vi "setStringValue.vi"(8 "error in (no error)":errorcluster, 10 "stringValue":string, 11 "xmlNode.lvclass in":refnum<class "xmlNode.lvclass">) -> (0 "error out":errorcluster, 3 "xmlNode.lvclass out":refnum<class "xmlNode.lvclass">)   [LabVIEW 2009, in "Tools.lvlib" / "xml.lvlib" / "xmlNode.lvclass"]
doc: "Sets the String value of an xml node\ni.e. sets \"value\" in this example\n\n<xml node> \"value\" </xml node>"
uses:
  xmlNode.lvclass
  xmlNode.lvclass/xmlNode.ctl
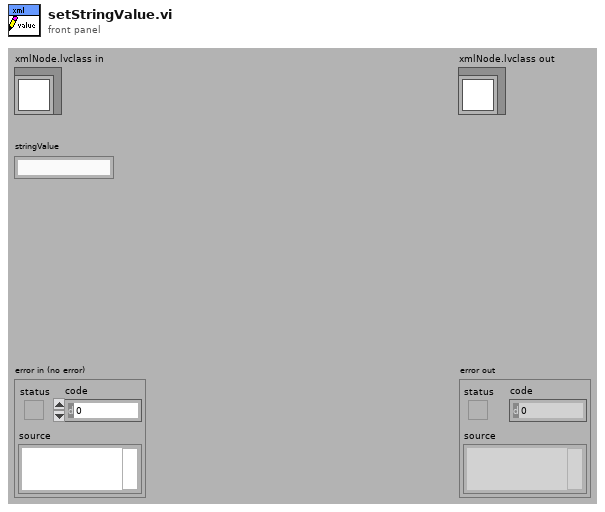
[diagram p1: front panel]
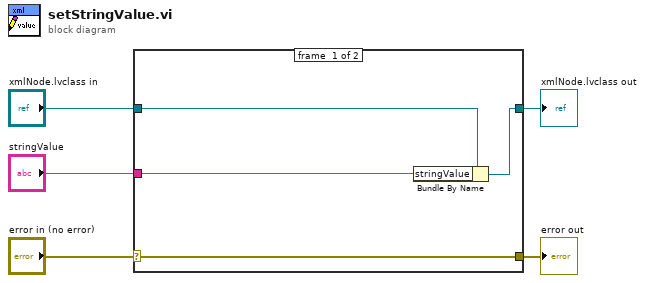
[diagram p0: block diagram]
diagram:
  n1 = case shown="No Error" "error in (no error)" {
    selector: "error in (no error)" -> [w9 w10]
    tunnel: [w9 w10] -> w4
    tunnel: [w7 w11] -> w2
    tunnel: "xmlNode.lvclass in" -> [w8 w11]
    tunnel: "stringValue" -> [w6 _]
    frame #0 {
      n2 = Bundle By Name(cluster=w8, "stringValue"=w6) -> (w7:refnum<class "xmlNode.lvclass">)
    }
    frame #1 {
    }
  }
  "error out" <- w4
  "xmlNode.lvclass out" <- w2
